vi "Module Loop.vi"(8 "error in (no error)":errorcluster, 11 "Telemetry Server Module in":refnum<class "Telemetry Server Module.lvclass">) -> (0 "error out":errorcluster, 3 "Telemetry Server Module out":refnum<class "Telemetry Server Module.lvclass">)   [LabVIEW 2020, in "Volatus.lvlib" / "Telemetry Server Module.lvclass"]
uses:
  Telemetry Server Module.lvclass
  Telemetry Server Module.lvclass/Telemetry Server Module.ctl
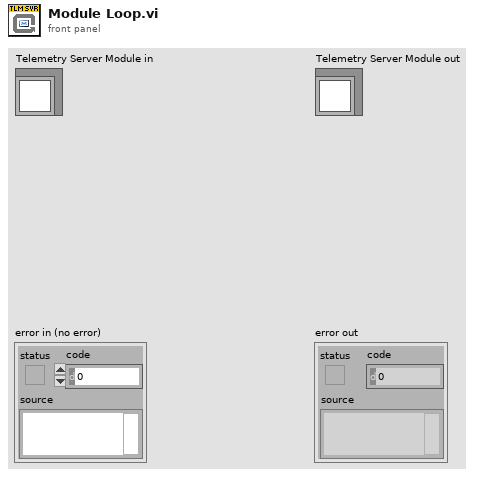
[diagram p1: front panel]
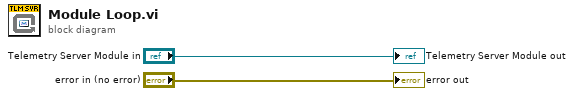
[diagram p0: block diagram]
diagram:
  "error out" <- "error in (no error)"
  "Telemetry Server Module out" <- "Telemetry Server Module in"
